vi "update image.vi"(7 "robot location":cluster{"x":i32, "y":i32, "direction":dbl}, 9 "menu":enum16{"Update", "Get", "Reset"}(ring), 10 "object":T2 {"direction" step=0.1}, 11 "raster image":T1[][](array[typedef])) -> ()   [LabVIEW 2009]
uses:
  object.ctl
  pixel 2.ctl
panel:
  out "raster image":T1[][](array[typedef])
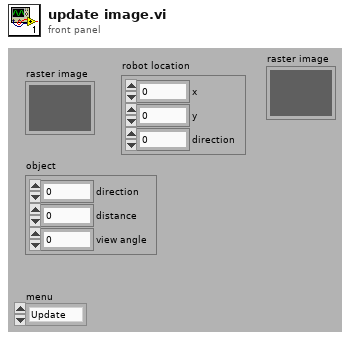
[diagram p1: front panel]
types:
  T1 = typedef "pixel 2.ctl" = bool
  T2 = typedef "object.ctl" = cluster{"direction":dbl, "distance":u32, "view angle":dbl}
  T3 = cluster{"left":i16, "top":i16, "right":i16, "bottom":i16}
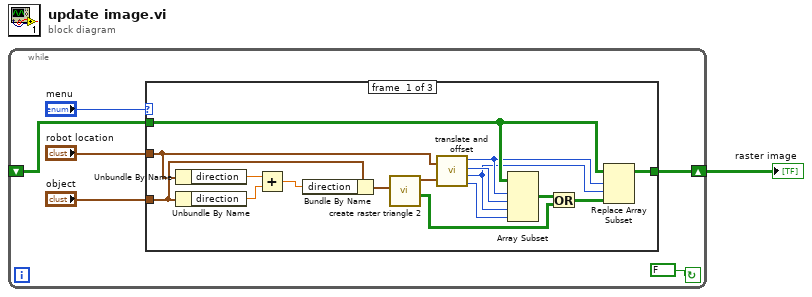
[diagram p0: block diagram]
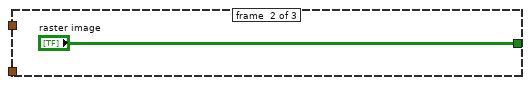
[diagram p2: hidden frame]
diagram:
  n1 = while {
    shift-right: [w5] -> w1
    shift-left: _ -> [w6]
    stop <- FALSE continue-if-true
    n2 = case shown="\"Update\"" "menu" {
      tunnel: "object" -> [w23 _ _]
      tunnel: "robot location" -> [w17 _ _]
      tunnel: w6 -> [w14 _ w25]
      tunnel: [w11 "raster image" w25] -> w5
      frame #0 {
        n3 = Unbundle By Name(w17) -> ("direction"=w21:dbl)
        n4 = Unbundle By Name(w23) -> ("direction"=w22:dbl)
        n5 = Add(x=w21, y=w22) -> (x+y=w20:dbl)
        n6 = Bundle By Name(cluster=w23, "direction"=w20) -> (w19:T2)
        n7 = call "create raster triangle 2.vi"("object"=w19) -> ("raster image"=w10:bool[][], "rect"=w18:T3)  [unwired: 9 in]
        n8 = call "translate and offset.vi"("robot location"=w17, "rect"=w18) -> ("index 0"=w13:i32, "length 0"=w16:i32, "index 1"=w12:i32, "length 1"=w15:i32)
        n9 = Array Subset(array=w14, index (row)=w13, length (row)=w16, index (col)=w12, length (col)=w15) -> (w9:T1[][])
        n10 = Or(x=w9, y=w10) -> (x .or. y?=w8:T1[][])
        n11 = Replace Array Subset(array=w14, new element=w8, index (row)=w13, index (col)=w12) -> (w11:T1[][])
      }
      frame #1 {
      }
      frame #2 {
      }
    }
  }
  "raster image" <- w1
